vi "example_RunningAllan_1.vi"() -> ()   [LabVIEW 2015]
uses:
  <vilib>/GPower/Array/Library/Create/Range/CreateRangeSGL.vi
  <vilib>/GPower/Array/Library/RemDup/RemDup_SGL.vi
  <vilib>/ptbypt/NI_PtbyPt.lvlib
  <vilib>/GPower/Array/GPArray.lvlib
panel:
  in  "stop":bool
  out "ok?":bool
  out "i":i32
  out "XY Graph":cluster{dbl[], "allanDevs":dbl[]}(graph)
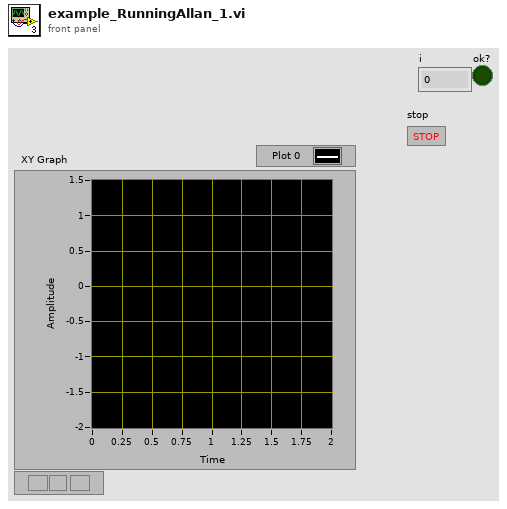
[diagram p1: front panel]
types:
  T1 = typedef "core_RunningAllanCarry.vi" = cluster{"lengths":i32[], "lengthsN":i32, "procL":i32[], "procI":i32[], "proc":dbl[], "procN":i32[], "allanDevsWIP":dbl[], "allanDevs":dbl[], "N":i32}
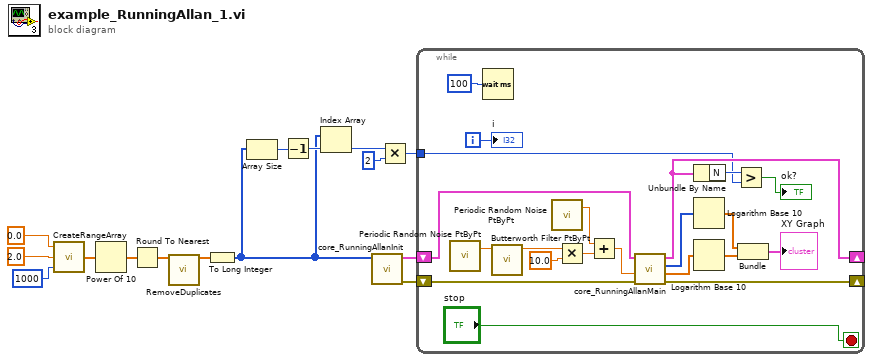
[diagram p0: block diagram]
diagram:
  n1 = call-poly <vilib>:"CreateRangeArray.vi"("N"=1000, "Range end"=sgl 2.0, "Range begin"=sgl 0.0) -> ("Created array"=w8:sgl[])
  n2 = Power Of 10(x=w8) -> (10^x=w7:sgl[])
  n3 = Round To Nearest(number=w7) -> (nearest integer value=w6:sgl[])
  n4 = call-poly <vilib>:"RemoveDuplicates.vi"("Array"=w6) -> ("Array with duplicates removed"=w5:sgl[])  [unwired: 12 in, 2 out]
  n5 = To Long Integer(number=w5) -> (32bit integer=w4:i32[])
  n6 = Array Size(array=w4) -> (size(s)=w13:i32)
  n7 = Decrement(x=w13) -> (x-1=w12:i32)
  n8 = Index Array(array=w4, index=w12) -> (element=w3:i32)
  n9 = call "core_RunningAllanInit.vi"("lengths"=w4) -> ("error out"=w14:errorcluster, "RACarry cluster"=w15:T1)  [unwired: 8 in, 1 out]
  n10 = Multiply(x=w3, y=2) -> (x*y=w2:i32)
  n11 = while {
    shift-right: [w34] -> _
    shift-left: w14 -> [w35]
    shift-right: [w31] -> _
    shift-left: w15 -> [w36]
    tunnel: w2 -> [w29]
    i -> [w23]
    stop <- "stop" stop-if-true
    n12 = call <vilib>:"Periodic Random Noise PtByPt.vi"() -> ("periodic random noise"=w22:dbl)  [unwired: 4 in, 1 out]
    n13 = Wait (ms)(milliseconds to wait=u32 100) -> ()  [unwired: 1 out]
    n14 = call <vilib>:"Butterworth Filter PtByPt.vi"("x"=w22) -> ("Filtered x"=w21:dbl)  [unwired: 8 in, 1 out]
    n15 = call <vilib>:"Periodic Random Noise PtByPt.vi"() -> ("periodic random noise"=w18:dbl)  [unwired: 4 in, 1 out]
    n16 = Multiply(x=w21, y=10.0) -> (x*y=w19:dbl)
    n17 = Add(x=w18, y=w19) -> (x+y=w17:dbl)
    n18 = call "core_RunningAllanMain.vi"("error in (no error)"=w35, "input data point"=w17, "RunningAllanCarry in"=w36) -> ("error out"=w34:errorcluster, "allanDevs"=w25:dbl[], "lengths"=w27:i32[], "RunningAllanCarry out"=w31:T1)  [unwired: 5 in]
    n19 = Unbundle By Name(w31) -> ("N"=w30:i32)
    n20 = Logarithm Base 10(1:w27) -> (0:w26:dbl[])
    n21 = Logarithm Base 10(1:w25) -> (0:w24:dbl[])
    n22 = Greater?(x=w30, y=w29) -> (0:→"ok?":bool)
    n23 = Bundle(w26, w24) -> (→"XY Graph":cluster{dbl[], dbl[]})  [unwired: 1 in]
    "i" <- w23
  }
